vi "XY Graph Get Plot Info & Clip Data.vi"(8 "error in (no error)":errorcluster, 9 "Clip Plot? (True)":bool=TRUE, 10 "Plot index":i32, 11 "XYGraph Ref in":refnum<vi>) -> (0 "error out":errorcluster, 1 "Y Array":dbl[](array[numeric]), 2 "X Array":dbl[](array[numeric]), 3 "XYGraph Ref out":refnum<vi>, 4 "Plot Name":string, 6 "Plot Color":u32)   [LabVIEW 2019]
panel:
  # "-1: last plot\n-2: next to last plot\n-3: etc..."
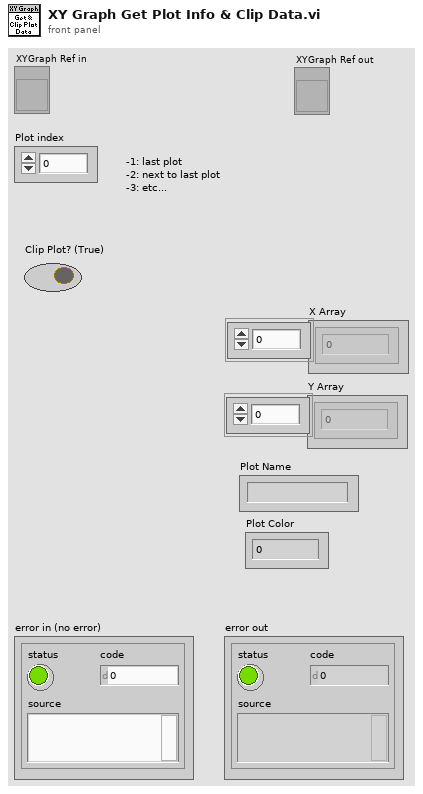
[diagram p1: front panel]
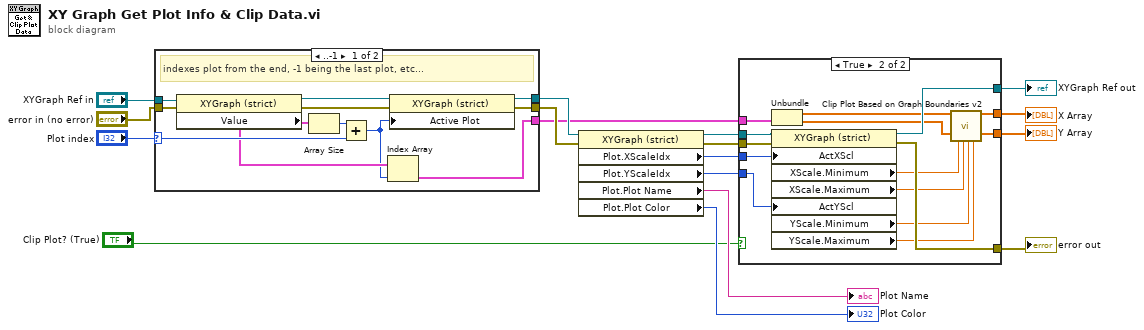
[diagram p0: block diagram]
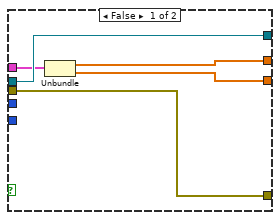
[diagram p2: hidden frame]
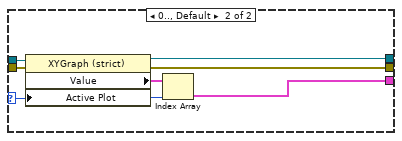
[diagram p3: hidden frame]
diagram:
  n1 = case shown="..-1" "Plot index" {
    selector: "Plot index" -> [w25 w30]
    tunnel: [w22 w34] -> w8
    tunnel: "XYGraph Ref in" -> [w28 w33]
    tunnel: "error in (no error)" -> [w27 w32]
    tunnel: [w21 w31] -> w5
    tunnel: [w18 w29] -> w3
    frame ..-1 {
      # "indexes plot from the end, -1 being the last plot, etc..."
      n2 = property class="XYGraph (strict)"(reference=w28, error in=w27) -> (reference out=w24:refnum<vi>, error out=w23:errorcluster, "Value"=w20:cluster{dbl[], dbl[]}[])
      n3 = Array Size(array=w20) -> (size(s)=w26:i32)
      n4 = Add(x=w26, y=w25) -> (x+y=w19:i32)
      n5 = Index Array(array=w20, index=w19) -> (element=w18:cluster{dbl[], dbl[]})
      n6 = property class="XYGraph (strict)"(reference=w24, error in=w23, "Active Plot"=w19) -> (reference out=w22:refnum<vi>, error out=w21:errorcluster)
    }
    frame 0.., Default {
      n7 = property class="XYGraph (strict)"(reference=w33, error in=w32, "Active Plot"=w30) -> (reference out=w34:refnum<vi>, error out=w31:errorcluster, "Value"=w35:cluster{dbl[], dbl[]}[])
      n8 = Index Array(array=w35, index=w30) -> (element=w29:cluster{dbl[], dbl[]})
    }
  }
  n9 = property class="XYGraph (strict)"(reference=w8, error in=w5) -> (reference out=w14:refnum<vi>, error out=w12:errorcluster, "Plot.XScaleIdx"=w10:u32, "Plot.YScaleIdx"=w9:u32, "Plot.Plot Name"=→"Plot Name":string, "Plot.Plot Color"=→"Plot Color":u32)
  n10 = case shown="True" "Clip Plot? (True)" {
    tunnel: w3 -> [w38 w49]
    tunnel: w14 -> [w40 w55]
    tunnel: [w40 w53] -> w13
    tunnel: w12 -> [w39 w54]
    tunnel: [w39 w52] -> w11
    tunnel: w10 -> [_ w51]
    tunnel: w9 -> [_ w50]
    tunnel: [w37 w46] -> w2
    tunnel: [w36 w45] -> w1
    frame False {
      n11 = Unbundle(w38) -> (w37:dbl[], w36:dbl[])
    }
    frame True {
      n12 = Unbundle(w49) -> (w48:dbl[], w47:dbl[])
      n13 = property class="XYGraph (strict)"(reference=w55, error in=w54, "ActXScl"=w51, "ActYScl"=w50) -> (reference out=w53:refnum<vi>, error out=w52:errorcluster, "XScale.Minimum"=w44:dbl, "XScale.Maximum"=w43:dbl, "YScale.Minimum"=w42:dbl, "YScale.Maximum"=w41:dbl)
      n14 = call "Clip Plot Based on Graph Boundaries v2.vi"("X Array in"=w48, "Y Array in"=w47, "XScale.Minimum (-Inf)"=w44, "XScale.Maximum (Inf)"=w43, "YScale.Minimum (-Inf)"=w42, "YScale.Maximum (Inf)"=w41) -> ("X Array out"=w46:dbl[], "Y Array out"=w45:dbl[])  [unwired: 12 in]
    }
  }
  "X Array" <- w2
  "Y Array" <- w1
  "XYGraph Ref out" <- w13
  "error out" <- w11
